vi "Delete Temporary vi.vi"(4 "Temporary File Created?":bool, 6 "File to Add":path, 8 "error in (no error)":errorcluster) -> (0 "error out":errorcluster)   [LabVIEW 2018]
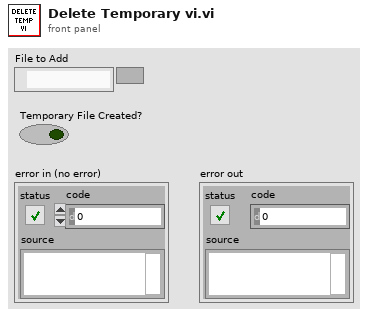
[diagram p1: front panel]
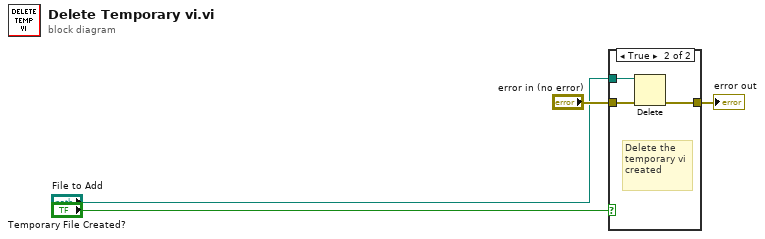
[diagram p0: block diagram]
diagram:
  n1 = case shown="True" "Temporary File Created?" {
    tunnel: "error in (no error)" -> [w5 w8]
    tunnel: [w5 w7] -> w1
    tunnel: "File to Add" -> [_ w6]
    frame False {
    }
    frame True {
      # "Delete the temporary vi created"
      n2 = Delete(path (use dialog)=w6, error in=w8) -> (error out=w7:errorcluster)  [unwired: 3 in, 2 out]
    }
  }
  "error out" <- w1
